vi "Main.vi"() -> ()   [LabVIEW 2018] (continued)
                n1556 = property on="102" class="Bool (严格)"("Colors [4]"=w7382) -> ()  [unwired: 2 in, 2 out]
                n1557 = property on="201" class="Bool (严格)"("Colors [4]"=w7382) -> ()  [unwired: 2 in, 2 out]
                n1558 = property on="301" class="Bool (严格)"("Colors [4]"=w7382) -> ()  [unwired: 2 in, 2 out]
                n1559 = property on="401" class="Bool (严格)"("Colors [4]"=w7382) -> ()  [unwired: 2 in, 2 out]
                n1560 = property on="501" class="Bool (严格)"("Colors [4]"=w7382) -> ()  [unwired: 2 in, 2 out]
                n1561 = property on="502" class="Bool (严格)"("Colors [4]"=w7382) -> ()  [unwired: 2 in, 2 out]
                n1562 = property on="503" class="Bool (严格)"("Colors [4]"=w7382) -> ()  [unwired: 2 in, 2 out]
                n1563 = property on="601" class="Bool (严格)"("Colors [4]"=w7382) -> ()  [unwired: 2 in, 2 out]
                n1564 = property on="70" class="Bool (严格)"("Colors [4]"=w7382) -> ()  [unwired: 2 in, 2 out]
                n1565 = property on="80" class="Bool (严格)"("Colors [4]"=w7382) -> ()  [unwired: 2 in, 2 out]
                n1566 = property on="901" class="Bool (严格)"("Colors [4]"=w7382) -> ()  [unwired: 2 in, 2 out]
                n1567 = property on="902" class="Bool (严格)"("Colors [4]"=w7382) -> ()  [unwired: 2 in, 2 out]
                n1568 = property on="602" class="Bool (严格)"("Colors [4]"=w7382) -> ()  [unwired: 2 in, 2 out]
                n1569 = property on="603" class="Bool (严格)"("Colors [4]"=w7382) -> ()  [unwired: 2 in, 2 out]
                n1570 = property on="202" class="Bool (严格)"("Colors [4]"=w7382) -> ()  [unwired: 2 in, 2 out]
                n1571 = property on="302" class="Bool (严格)"("Colors [4]"=w7382) -> ()  [unwired: 2 in, 2 out]
                n1572 = property on="303" class="Bool (严格)"("Colors [4]"=w7382) -> ()  [unwired: 2 in, 2 out]
                n1573 = property on="402" class="Bool (严格)"("Colors [4]"=w7382) -> ()  [unwired: 2 in, 2 out]
                n1574 = property on="504" class="Bool (严格)"("Colors [4]"=w7382) -> ()  [unwired: 2 in, 2 out]
              }
              frame #1 {
                n1575 = Concatenate Strings("Where QRCode='" ("查询语句"), "输入需要Rework的一维码：", "'" ("字符串")) -> (w7412:string)
                n1576 = call "SQL_Select.vi"("要读取的列名"=string[] ["Last_Station", "Last_Result"] ("列名"), "表名"="Online", "error in (no error)"=w7410, "查询语句"=w7412, "查询条件"=TRUE, "connection reference"=w7411) -> ("error out"=w7402:errorcluster, "数据"=w7407:string[][])  [unwired: 3 in, 1 out]
                n1577 = Index Array(array=w7407, index (row)=0 ("索引 (行)")) -> (element=w7405:string[])  [unwired: 1 in]
                n1578 = Index Array(array=w7405) -> (element #1=w7404:string, element #2=w7403:string)  [unwired: 2 in]
                n1579 = case shown="\"902\"" w7404 {
                  tunnel: [w7417 w7419 TRUE w7432 w7439 w7446 w7453 w7460 w7467 w7474 w7481 w7488 w7495 w7502 w7509 w7516 w7523 w7530 w7537 w7543] -> w7401
                  tunnel: [w7417 w7418 w7426 w7432 w7439 w7446 w7453 w7460 w7467 w7474 w7481 w7488 w7495 w7502 w7509 w7516 w7523 w7530 w7537 w7543] -> w7400
                  tunnel: [w7417 w7418 w7424 w7433 w7439 w7446 w7453 w7460 w7467 w7474 w7481 w7488 w7495 w7502 w7509 w7516 w7523 w7530 w7537 w7543] -> w7399
                  tunnel: [w7417 w7418 w7424 w7431 w7440 w7446 w7453 w7460 w7467 w7474 w7481 w7488 w7495 w7502 w7509 w7516 w7523 w7530 w7537 w7543] -> w7398
                  tunnel: [w7417 w7418 w7424 w7431 w7438 w7447 w7453 w7460 w7467 w7474 w7481 w7488 w7495 w7502 w7509 w7516 w7523 w7530 w7537 w7543] -> w7397
                  tunnel: [w7417 w7418 w7424 w7431 w7438 w7445 w7454 w7460 w7467 w7474 w7481 w7488 w7495 w7502 w7509 w7516 w7523 w7530 w7537 w7543] -> w7396
                  tunnel: [w7417 w7418 w7424 w7431 w7438 w7445 w7452 w7461 w7467 w7474 w7481 w7488 w7495 w7502 w7509 w7516 w7523 w7530 w7537 w7543] -> w7395
                  tunnel: [w7417 w7418 w7424 w7431 w7438 w7445 w7452 w7459 w7468 w7474 w7481 w7488 w7495 w7502 w7509 w7516 w7523 w7530 w7537 w7543] -> w7394
                  tunnel: [w7417 w7418 w7424 w7431 w7438 w7445 w7452 w7459 w7466 w7475 w7481 w7488 w7495 w7502 w7509 w7516 w7523 w7530 w7537 w7543] -> w7393
                  tunnel: [w7417 w7418 w7424 w7431 w7438 w7445 w7452 w7459 w7466 w7473 w7483 w7488 w7495 w7502 w7509 w7516 w7523 w7530 w7537 w7543] -> w7392
                  tunnel: [w7417 w7418 w7424 w7431 w7438 w7445 w7452 w7459 w7466 w7473 w7480 w7490 w7495 w7502 w7509 w7516 w7523 w7530 w7537 w7543] -> w7391
                  tunnel: [w7417 w7418 w7424 w7431 w7438 w7445 w7452 w7459 w7466 w7473 w7480 w7487 w7496 w7502 w7509 w7516 w7523 w7530 w7537 w7543] -> w7390
                  tunnel: [w7417 w7418 w7424 w7431 w7438 w7445 w7452 w7459 w7466 w7473 w7480 w7487 w7494 w7504 w7509 w7516 w7523 w7530 w7537 w7543] -> w7389
                  tunnel: [w7417 w7418 w7424 w7431 w7438 w7445 w7452 w7459 w7466 w7473 w7480 w7487 w7494 w7501 w7510 w7516 w7523 w7530 w7537 w7543] -> w7388
                  tunnel: [w7417 w7418 w7424 w7431 w7438 w7445 w7452 w7459 w7466 w7473 w7480 w7487 w7494 w7501 w7508 w7517 w7523 w7530 w7537 w7543] -> w7387
                  tunnel: [w7417 w7418 w7424 w7431 w7438 w7445 w7452 w7459 w7466 w7473 w7480 w7487 w7494 w7501 w7508 w7515 w7524 w7530 w7537 w7543] -> w7386
                  tunnel: [w7417 w7418 w7424 w7431 w7438 w7445 w7452 w7459 w7466 w7473 w7480 w7487 w7494 w7501 w7508 w7515 w7522 w7531 w7537 w7543] -> w7385
                  tunnel: [w7417 w7418 w7424 w7431 w7438 w7445 w7452 w7459 w7466 w7473 w7480 w7487 w7494 w7501 w7508 w7515 w7522 w7529 w7539 w7543] -> w7384
                  tunnel: [w7417 w7418 w7424 w7431 w7438 w7445 w7452 w7459 w7466 w7473 w7480 w7487 w7494 w7501 w7508 w7515 w7522 w7529 FALSE w7545] -> w7383
                  tunnel: w7403 -> [_ w7420 w7427 w7434 w7441 w7448 w7455 w7462 w7469 w7476 w7482 w7489 w7497 w7503 w7511 w7518 w7525 w7532 w7538 w7544]
                  frame "0", Default {
                    w7417 = FALSE
                  }
                  frame "102" {
                    w7418 = FALSE
                    n1580 = case shown="\"NG\"" w7420 {
                      tunnel: [TRUE FALSE] -> w7419
                      frame "OK", Default {
                      }
                      frame "NG" {
                        n1581 = property on="102" class="Bool (严格)"("Colors [4]"=cluster{u32, u32}[] [{16711680, 16711680}, {6618880, 6618880}, {1985280, 1985280}, {6618880, 6618880}] ("颜色[4]")) -> ()  [unwired: 2 in, 2 out]
                      }
                    }
                  }
                  frame "201" {
                    w7424 = FALSE
                    n1582 = case shown="\"NG\"" w7427 {
                      tunnel: [TRUE FALSE] -> w7426
                      frame "OK", Default {
                      }
                      frame "NG" {
                        n1583 = property on="201" class="Bool (严格)"("Colors [4]"=cluster{u32, u32}[] [{16711680, 16711680}, {6618880, 6618880}, {1985280, 1985280}, {6618880, 6618880}] ("颜色[4]")) -> ()  [unwired: 2 in, 2 out]
                      }
                    }
                  }
                  frame "202" {
                    w7432 = TRUE
                    w7431 = FALSE
                    n1584 = case shown="\"NG\"" w7434 {
                      tunnel: [TRUE FALSE] -> w7433
                      frame "OK", Default {
                      }
                      frame "NG" {
                        n1585 = property on="202" class="Bool (严格)"("Colors [4]"=cluster{u32, u32}[] [{16711680, 16711680}, {6618880, 6618880}, {1985280, 1985280}, {6618880, 6618880}] ("颜色[4]")) -> ()  [unwired: 2 in, 2 out]
                      }
                    }
                  }
                  frame "301" {
                    w7438 = FALSE
                    w7439 = TRUE
                    n1586 = case shown="\"NG\"" w7441 {
                      tunnel: [TRUE FALSE] -> w7440
                      frame "OK", Default {
                      }
                      frame "NG" {
                        n1587 = property on="301" class="Bool (严格)"("Colors [4]"=cluster{u32, u32}[] [{16711680, 16711680}, {6618880, 6618880}, {1985280, 1985280}, {6618880, 6618880}] ("颜色[4]")) -> ()  [unwired: 2 in, 2 out]
                      }
                    }
                  }
                  frame "302" {
                    w7445 = FALSE
                    w7446 = TRUE
                    n1588 = case shown="\"NG\"" w7448 {
                      tunnel: [TRUE FALSE] -> w7447
                      frame "OK", Default {
                      }
                      frame "NG" {
                        n1589 = property on="302" class="Bool (严格)"("Colors [4]"=cluster{u32, u32}[] [{16711680, 16711680}, {6618880, 6618880}, {1985280, 1985280}, {6618880, 6618880}] ("颜色[4]")) -> ()  [unwired: 2 in, 2 out]
                      }
                    }
                  }
                  frame "303" {
                    w7452 = FALSE
                    w7453 = TRUE
                    n1590 = case shown="\"NG\"" w7455 {
                      tunnel: [TRUE FALSE] -> w7454
                      frame "OK", Default {
                      }
                      frame "NG" {
                        n1591 = property on="303" class="Bool (严格)"("Colors [4]"=cluster{u32, u32}[] [{16711680, 16711680}, {6618880, 6618880}, {1985280, 1985280}, {6618880, 6618880}] ("颜色[4]")) -> ()  [unwired: 2 in, 2 out]
                      }
                    }
                  }
                  frame "401" {
                    w7459 = FALSE
                    w7460 = TRUE
                    n1592 = case shown="\"NG\"" w7462 {
                      tunnel: [TRUE FALSE] -> w7461
                      frame "OK", Default {
                      }
                      frame "NG" {
                        n1593 = property on="401" class="Bool (严格)"("Colors [4]"=cluster{u32, u32}[] [{16711680, 16711680}, {6618880, 6618880}, {1985280, 1985280}, {6618880, 6618880}] ("颜色[4]")) -> ()  [unwired: 2 in, 2 out]
                      }
                    }
                  }
                  frame "402" {
                    w7466 = FALSE
                    w7467 = TRUE
                    n1594 = case shown="\"NG\"" w7469 {
                      tunnel: [TRUE FALSE] -> w7468
                      frame "OK", Default {
                      }
                      frame "NG" {
                        n1595 = property on="402" class="Bool (严格)"("Colors [4]"=cluster{u32, u32}[] [{16711680, 16711680}, {6618880, 6618880}, {1985280, 1985280}, {6618880, 6618880}] ("颜色[4]")) -> ()  [unwired: 2 in, 2 out]
                      }
                    }
                  }
                  frame "501" {
                    w7473 = FALSE
                    w7474 = TRUE
                    n1596 = case shown="\"NG\"" w7476 {
                      tunnel: [TRUE FALSE] -> w7475
                      frame "OK", Default {
                      }
                      frame "NG" {
                        n1597 = property on="501" class="Bool (严格)"("Colors [4]"=cluster{u32, u32}[] [{16711680, 16711680}, {6618880, 6618880}, {1985280, 1985280}, {6618880, 6618880}] ("颜色[4]")) -> ()  [unwired: 2 in, 2 out]
                      }
                    }
                  }
                  frame "502" {
                    w7480 = FALSE
                    w7481 = TRUE
                    n1598 = case shown="\"NG\"" w7482 {
                      tunnel: [TRUE FALSE] -> w7483
                      frame "OK", Default {
                      }
                      frame "NG" {
                        n1599 = property on="502" class="Bool (严格)"("Colors [4]"=cluster{u32, u32}[] [{16711680, 16711680}, {6618880, 6618880}, {1985280, 1985280}, {6618880, 6618880}] ("颜色[4]")) -> ()  [unwired: 2 in, 2 out]
                      }
                    }
                  }
                  frame "503" {
                    w7487 = FALSE
                    w7488 = TRUE
                    n1600 = case shown="\"NG\"" w7489 {
                      tunnel: [TRUE FALSE] -> w7490
                      frame "OK", Default {
                      }
                      frame "NG" {
                        n1601 = property on="503" class="Bool (严格)"("Colors [4]"=cluster{u32, u32}[] [{16711680, 16711680}, {6618880, 6618880}, {1985280, 1985280}, {6618880, 6618880}] ("颜色[4]")) -> ()  [unwired: 2 in, 2 out]
                      }
                    }
                  }
                  frame "504" {
                    w7494 = FALSE
                    w7495 = TRUE
                    n1602 = case shown="\"NG\"" w7497 {
                      tunnel: [TRUE FALSE] -> w7496
                      frame "OK", Default {
                      }
                      frame "NG" {
                        n1603 = property on="504" class="Bool (严格)"("Colors [4]"=cluster{u32, u32}[] [{16711680, 16711680}, {6618880, 6618880}, {1985280, 1985280}, {6618880, 6618880}] ("颜色[4]")) -> ()  [unwired: 2 in, 2 out]
                      }
                    }
                  }
                  frame "601" {
                    w7501 = FALSE
                    w7502 = TRUE
                    n1604 = case shown="\"NG\"" w7503 {
                      tunnel: [TRUE FALSE] -> w7504
                      frame "OK", Default {
                      }
                      frame "NG" {
                        n1605 = property on="601" class="Bool (严格)"("Colors [4]"=cluster{u32, u32}[] [{16711680, 16711680}, {6618880, 6618880}, {1985280, 1985280}, {6618880, 6618880}] ("颜色[4]")) -> ()  [unwired: 2 in, 2 out]
                      }
                    }
                  }
                  frame "602" {
                    w7508 = FALSE
                    w7509 = TRUE
                    n1606 = case shown="\"NG\"" w7511 {
                      tunnel: [TRUE FALSE] -> w7510
                      frame "OK", Default {
                      }
                      frame "NG" {
                        n1607 = property on="602" class="Bool (严格)"("Colors [4]"=cluster{u32, u32}[] [{16711680, 16711680}, {6618880, 6618880}, {1985280, 1985280}, {6618880, 6618880}] ("颜色[4]")) -> ()  [unwired: 2 in, 2 out]
                      }
                    }
                  }
                  frame "603" {
                    w7515 = FALSE
                    w7516 = TRUE
                    n1608 = case shown="\"NG\"" w7518 {
                      tunnel: [TRUE FALSE] -> w7517
                      frame "OK", Default {
                      }
                      frame "NG" {
                        n1609 = property on="603" class="Bool (严格)"("Colors [4]"=cluster{u32, u32}[] [{16711680, 16711680}, {6618880, 6618880}, {1985280, 1985280}, {6618880, 6618880}] ("颜色[4]")) -> ()  [unwired: 2 in, 2 out]
                      }
                    }
                  }
                  frame "70" {
                    w7522 = FALSE
                    w7523 = TRUE
                    n1610 = case shown="\"NG\"" w7525 {
                      tunnel: [TRUE FALSE] -> w7524
                      frame "OK", Default {
                      }
                      frame "NG" {
                        n1611 = property on="70" class="Bool (严格)"("Colors [4]"=cluster{u32, u32}[] [{16711680, 16711680}, {6618880, 6618880}, {1985280, 1985280}, {6618880, 6618880}] ("颜色[4]")) -> ()  [unwired: 2 in, 2 out]
                      }
                    }
                  }
                  frame "80" {
                    w7529 = FALSE
                    w7530 = TRUE
                    n1612 = case shown="\"NG\"" w7532 {
                      tunnel: [TRUE FALSE] -> w7531
                      frame "OK", Default {
                      }
                      frame "NG" {
                        n1613 = property on="80" class="Bool (严格)"("Colors [4]"=cluster{u32, u32}[] [{16711680, 16711680}, {6618880, 6618880}, {1985280, 1985280}, {6618880, 6618880}] ("颜色[4]")) -> ()  [unwired: 2 in, 2 out]
                      }
                    }
                  }
                  frame "901" {
                    w7537 = TRUE
                    n1614 = case shown="\"OK\", 默认" w7538 {
                      tunnel: [TRUE FALSE] -> w7539
                      frame "OK", Default {
                      }
                      frame "NG" {
                        n1615 = property on="901" class="Bool (严格)"("Colors [4]"=cluster{u32, u32}[] [{16711680, 16711680}, {6618880, 6618880}, {1985280, 1985280}, {6618880, 6618880}] ("颜色[4]")) -> ()  [unwired: 2 in, 2 out]
                      }
                    }
                  }
                  frame "902" {
                    w7543 = TRUE
                    n1616 = case shown="\"NG\"" w7544 {
                      tunnel: [TRUE FALSE] -> w7545
                      frame "OK", Default {
                      }
                      frame "NG" {
                        n1617 = property on="902" class="Bool (严格)"("Colors [4]"=cluster{u32, u32}[] [{16711680, 16711680}, {6618880, 6618880}, {1985280, 1985280}, {6618880, 6618880}] ("颜色[4]")) -> ()  [unwired: 2 in, 2 out]
                      }
                    }
                  }
                }
                n1618 = local write "102"(w7401) -> ()
                n1619 = local write "201"(w7400) -> ()
                n1620 = local write "202"(w7399) -> ()
                n1621 = local write "301"(w7398) -> ()
                n1622 = local write "302"(w7397) -> ()
                n1623 = local write "303"(w7396) -> ()
                n1624 = local write "401"(w7395) -> ()
                n1625 = local write "402"(w7394) -> ()
                n1626 = local write "501"(w7393) -> ()
                n1627 = local write "502"(w7392) -> ()
                n1628 = local write "503"(w7391) -> ()
                n1629 = local write "504"(w7390) -> ()
                n1630 = local write "601"(w7389) -> ()
                n1631 = local write "602"(w7388) -> ()
                n1632 = local write "603"(w7387) -> ()
                n1633 = local write "70"(w7386) -> ()
                n1634 = local write "80"(w7385) -> ()
                n1635 = local write "901"(w7384) -> ()
                n1636 = local write "902"(w7383) -> ()
              }
            }
          }
          event "确定Rework": Value Change {
            n1637 = event-data() -> ()  [unwired: 1 in, 2 out]
            n1638 = stacked-sequence {
              seq-local: [w7553 _] -> [_ w7586]
              tunnel: w7552 -> [w7563 w7591]
              tunnel: w7551 -> [w7562 w7590]
              tunnel: [_ w7589] -> w7550
              frame #0 {
                n1639 = local read "输入需要Rework的一维码："() -> (w7558:string)
                n1640 = Concatenate Strings("Where QRCode='" ("查询语句"), w7558, "'" ("字符串")) -> (w7557:string)
                n1641 = call "SQL_Select.vi"("表名"="Online", "error in (no error)"=w7562, "查询语句"=w7557, "查询条件"=TRUE, "connection reference"=w7563) -> ("数据"=w7556:string[][])  [unwired: 4 in, 2 out]
                n1642 = Matrix Size(0:w7556) -> (1:w7555:i32)  [unwired: 1 out]
                n1643 = Equal?(x=w7555, y=0) -> (x = y?=w7553:bool)
              }
              frame #1 {
                n1644 = Insert Into Array(array=bool[] [] ("数组"), index=0 ("索引"), new element #1="902", new element #2="901", new element #3="80", new element #4="70", new element #5="603", new element #6="602", new element #7="601", new element #8="504", new element #9="503", new element #10="502", new element #11="501", new element #12="402", new element #13="401", new element #14="303", new element #15="302", new element #16="301", new element #17="202", new element #18="201", new element #19="102") -> (w7595:bool[])
                n1645 = Search 1D Array(1D array=w7595, element=TRUE ("元素")) -> (index of element=w7592:i32)  [unwired: 1 in]
                n1646 = Equal?(x=w7592, y=-1) -> (x = y?=w7588:bool)
                n1647 = Or(x=w7588, y=w7586) -> (x .or. y?=w7587:bool)
                n1648 = case shown="假" w7587 {
                  tunnel: w7592 -> [w7637 _]
                  tunnel: w7591 -> [w7636 _]
                  tunnel: w7590 -> [w7635 w7754]
                  tunnel: [w7597 w7754] -> w7589
                  frame False {
                    w7609 = "Rework_List" ("表名")
                    w7607 = 0 ("索引 (行)")
                    w7620 = "Online" ("表名")
                    n1649 = case shown="8" w7637 {
                      tunnel: w7636 -> [w7698 w7700 w7704 w7707 w7710 w7713 w7716 w7719 w7722 w7725 w7728 w7731 w7733 w7736 w7739 w7742 w7745 w7748 w7751]
                      tunnel: w7635 -> [w7697 w7699 w7703 w7706 w7709 w7712 w7715 w7718 w7721 w7724 w7727 w7730 w7732 w7735 w7738 w7741 w7744 w7747 w7750]
                      tunnel: [w7697 w7699 w7703 w7706 w7709 w7712 w7715 w7718 w7721 w7724 w7727 w7730 w7732 w7735 w7738 w7741 w7744 w7747 w7750] -> w7623
                      tunnel: [w7698 w7700 w7704 w7707 w7710 w7713 w7716 w7719 w7722 w7725 w7728 w7731 w7733 w7736 w7739 w7742 w7745 w7748 w7751] -> w7624
                      tunnel: ["902" "901" "80" "70" "603" "602" "601" "504" "503" "502" "501" "402" "401" "303" "302" "301" "202" "201" "102"] -> w7604
                      frame 0, Default {
                      }
                      frame 1 {
                      }
                      frame 2 {
                      }
                      frame 3 {
                      }
                      frame 4 {
                      }
                      frame 5 {
                      }
                      frame 6 {
                      }
                      frame 7 {
                      }
                      frame 8 {
                      }
                      frame 9 {
                      }
                      frame 10 {
                      }
                      frame 11 {
                      }
                      frame 12 {
                      }
                      frame 13 {
                      }
                      frame 14 {
                      }
                      frame 15 {
                      }
                      frame 16 {
                      }
                      frame 17 {
                      }
                      frame 18 {
                      }
                    }
                    n1650 = local read "输入需要Rework的一维码："() -> (w7599:string)
                    n1651 = Concatenate Strings("Where QRCode='" ("查询语句"), w7599, "'" ("字符串")) -> (w7606:string)
                    n1652 = call "SQL_Select.vi"("要读取的列名"=string[] ["Last_Station"], "表名"=w7620, "error in (no error)"=w7623, "查询语句"=w7606, "查询条件"=TRUE, "connection reference"=w7624) -> ("error out"=w7621:errorcluster, "数据"=w7596:string[][], "connection reference out"=w7622:T5)  [unwired: 3 in]
                    n1653 = Index Array(array=w7596, index (row)=w7607, index (col)=w7607) -> (element=w7605:string)
                    n1654 = Insert Into Array(array=string[] [] ("数组"), index=0 ("索引"), new element #1=w7604, new element #2="OK" ("新元素/子数组"), new element #3="T" ("新元素/子数组")) -> (w7633:string[])
                    n1655 = call "SQL_Update.vi"("查询语句"=w7606, "表名"=w7620, "error in (no error)"=w7621, "列名对应的值"=w7633, "列名"=string[] ["Last_Station", "Last_Result", "Rework_Status"], "connection reference"=w7622) -> ("error out"=w7619:errorcluster, "connection reference 2"=w7618:T5)  [unwired: 4 in]
                    n1656 = call "SQL_Select.vi"("表名"=w7609, "error in (no error)"=w7619, "查询语句"=w7606, "查询条件"=TRUE, "connection reference"=w7618) -> ("error out"=w7612:errorcluster, "数据"=w7616:string[][], "connection reference out"=w7613:T5)  [unwired: 4 in]
                    n1657 = Matrix Size(0:w7616) -> (1:w7615:i32)  [unwired: 1 out]
                    n1658 = call "Rework_Calculate.vi"("Rework站号"=w7604, "当前站号"=w7605) -> ("Data"=w7611:string[], "Rework_List"=w7610:string[], "跨站"=w7603:bool)  [unwired: 7 in]
                    n1659 = Equal To 0?(x=w7615) -> (x = 0?=w7614:bool)
                    n1660 = case shown="假" w7603 {
                      tunnel: w7614 -> [w7656 _]
                      tunnel: w7613 -> [w7655 w7692]
                      tunnel: w7612 -> [w7654 w7693]
                      tunnel: w7611 -> [w7653 _]
                      tunnel: w7610 -> [w7652 _]
                      tunnel: w7609 -> [w7651 _]
                      tunnel: w7606 -> [w7647 _]
                      tunnel: w7599 -> [w7640 _]
                      tunnel: [w7639 w7693] -> w7601
                      tunnel: [w7638 w7692] -> w7602
                      frame False {
                        w7641 = "Rework" ("表名")
                        n1661 = case shown="真" w7656 {
                          tunnel: w7655 -> [w7678 w7691]
                          tunnel: w7654 -> [w7677 w7690]
                          tunnel: w7653 -> [w7675 w7685]
                          tunnel: w7652 -> [w7676 w7688]
                          tunnel: w7651 -> [w7674 w7689]
                          tunnel: w7640 -> [_ w7683]
                          tunnel: [w7672 w7680] -> w7649
                          tunnel: [w7671 w7679] -> w7648
                          tunnel: w7647 -> [w7673 _]
                          frame False {
                            n1662 = call "SQL_Update.vi"("查询语句"=w7673, "表名"=w7674, "error in (no error)"=w7677, "列名对应的值"=w7675, "列名"=w7676, "connection reference"=w7678) -> ("error out"=w7671:errorcluster, "connection reference 2"=w7672:T5)  [unwired: 4 in]
                          }
                          frame True {
                            n1663 = Insert Into Array(array=w7688, index=0 ("索引"), new element="QRCode" ("新元素/子数组")) -> (w7682:string[])
                            n1664 = Insert Into Array(array=w7685, index=0 ("索引"), new element=w7683) -> (w7681:string[])
                            n1665 = call "SQL_Insert.vi"("表名"=w7689, "error in (no error)"=w7690, "值"=w7681, "列名"=w7682, "connection reference"=w7691) -> ("error out"=w7679:errorcluster, "connection reference 2"=w7680:T5)  [unwired: 5 in]
                          }
                        }
                        n1666 = call "SQL_Select.vi"("表名"=w7641, "error in (no error)"=w7648, "查询语句"=w7647, "查询条件"=TRUE, "connection reference"=w7649) -> ("error out"=w7642:errorcluster, "数据"=w7646:string[][], "connection reference out"=w7643:T5)  [unwired: 4 in]
                        n1667 = Matrix Size(0:w7646) -> (1:w7645:i32)  [unwired: 1 out]
                        n1668 = Equal To 0?(x=w7645) -> (x = 0?=w7644:bool)
                        n1669 = case shown="真" w7644 {
                          tunnel: w7643 -> [w7657 w7670]
                          tunnel: w7642 -> [w7658 w7669]
                          tunnel: w7641 -> [_ w7668]
                          tunnel: w7640 -> [_ w7666]
                          tunnel: [w7658 w7662] -> w7639
                          tunnel: [w7657 w7659] -> w7638
                          frame False {
                          }
                          frame True {
                            n1670 = Format Date/Time String(time format string (%c)="%Y-%m-%d_%H:%M" ("时间格式字符串(%c)")) -> (date/time string=w7660:string)  [unwired: 2 in]
                            n1671 = Insert Into Array(array=string[] [] ("数组"), index=0 ("索引"), new element #1=w7666, new element #2=w7660) -> (w7663:string[])
                            n1672 = call "SQL_Insert.vi"("表名"=w7668, "error in (no error)"=w7669, "值"=w7663, "列名"=string[] ["QRCode", "Online_Time"], "connection reference"=w7670) -> ("error out"=w7662:errorcluster, "connection reference 2"=w7659:T5)  [unwired: 5 in]
                          }
                        }
                      }
                      frame True {
                      }
                    }
                    n1673 = call "SQL_Delete.vi"("表名"="Time", "error in (no error)"=w7601, "值"=w7599, "列名"="QRCode", "connection reference"=w7602) -> ("error out"=w7597:errorcluster)  [unwired: 5 in, 1 out]
                    n1674 = case shown="错误" w7597 {
                      tunnel: ["Rework成功！" ("Rework状态") "Rework失败！" ("Rework状态")] -> w7608
                      frame No Error {
                      }
                      frame Error {
                      }
                    }
                    "Rework状态" <- w7608
                  }
                  frame True {
                    n1675 = local write "Rework状态"("该条码不存在！" ("Rework状态")) -> ()
                  }
                }
              }
            }
          }
        }
        n1676 = case shown="错误" w4418 {
          selector: w4418 -> [_ w4425]
          tunnel: w4417 -> [_ w4430]
          frame No Error {
          }
          frame Error {
            n1677 = Unbundle By Name(w4425) -> ("source"=w4424:string)
            n1678 = property on="错误信息" class="LstBox (严格)"() -> ("Item Names"=w4429:string[])  [unwired: 2 in, 2 out]
            n1679 = Format Date/Time String(time format string (%c)="%Y-%m-%d %H:%M:%S" ("时间格式字符串(%c)")) -> (date/time string=w4432:string)  [unwired: 2 in]
            n1680 = Concatenate Strings(w4432, "  " ("字符串"), w4430, w4424) -> (w4427:string)
            n1681 = Insert Into Array(array=w4429, index=0 ("索引"), new element=w4427) -> (w4426:string[])
            n1682 = property on="错误信息" class="LstBox (严格)"("Item Names"=w4426) -> ()  [unwired: 2 in, 2 out]
          }
        }
        n1683 = local read "退出"() -> (w4419:bool)
        n1684 = Wait (ms)(milliseconds to wait=u32 30 ("等待时间（毫秒）")) -> ()  [unwired: 1 out]
      }
      n1685 = while {
        shift-right: [w4049] -> _
        shift-left: errorcluster {"status"=FALSE, "code"=0, "source"=""} ("错误常量") -> [w4052]
        shift-right: [w4048] -> _
        shift-left: enum16{"初始化", "读", "写", "错误", "退出"}."初始化" -> [w4054]
        shift-right: [w4050] -> _
        shift-left: _ -> [w4046]
        stop <- w4047 stop-if-true
        # "原100"
        n1686 = local read "退出"() -> (w4055:bool)
        n1687 = case shown="假" w4055 {
          tunnel: w4054 -> [w4056 _]
          tunnel: [w4057 enum16{"初始化", "读", "写", "错误", "退出"}."退出"] -> w4053
          tunnel: w4052 -> [w4058 _]
          frame False {
            n1688 = case shown="错误" w4058 {
              tunnel: [w4059 enum16{"初始化", "读", "写", "错误", "退出"}."错误"] -> w4057
              tunnel: w4056 -> [w4059 _]
              frame No Error {
              }
              frame Error {
              }
            }
          }
          frame True {
          }
        }
        n1689 = Wait (ms)(milliseconds to wait=u32 20 ("等待时间（毫秒）")) -> ()  [unwired: 1 out]
        n1690 = case shown="\"写\"" w4053 {
          tunnel: [w4065 w4104 w4311 refnum<k5> refnum ("TCP") refnum<k5> refnum ("TCP")] -> w4050
          tunnel: [w4063 w4103 w4313 errorcluster {"status"=FALSE, "code"=0, "source"=""} ("error out") errorcluster {"status"=FALSE, "code"=0, "source"=""} ("error out")] -> w4049
          tunnel: [enum16{"初始化", "读", "写", "错误", "退出"}."读" enum16{"初始化", "读", "写", "错误", "退出"}."写" enum16{"初始化", "读", "写", "错误", "退出"}."读" enum16{"初始化", "读", "写", "错误", "退出"}."初始化" enum16{"初始化", "读", "写", "错误", "退出"}."退出"] -> w4048
          tunnel: w4046 -> [_ w4145 w4342 w4407 w4414]
          tunnel: [FALSE FALSE FALSE FALSE TRUE] -> w4047
          frame "初始化", Default {
            w4066 = u16 0 items=["byte", "word", "Dword"] ("数据类型")
            w4068 = u8 132 items=["I/O (P)"=128, "Input (I)"=129, "Output (Q)"=130, "Bit Memory (M)"=131, "Data (DB)"=132, "Instance Data (DI)"=133, "Local Data (L)"=134, "Predecessor Local Data (VL)"=135] ("寄存器类型")
            w4082 = u16 0 items=["byte", "word", "Dword"] ("数据类型")
            w4084 = u8 132 items=["I/O (P)"=128, "Input (I)"=129, "Output (Q)"=130, "Bit Memory (M)"=131, "Data (DB)"=132, "Instance Data (DI)"=133, "Local Data (L)"=134, "Predecessor Local Data (VL)"=135] ("寄存器类型")
            w4091 = u8 0 items=["S7-1200.200.200SMART"=0, "S7-300"=2, "S7-400"=3] ("PLC 系列")
            n1691 = call "S7_Open.vi"("IP 地址"="192.168.1.10", "PLC 系列"=w4091, "超时（MS）"=100) -> ("TCP"=w4081:refnum<k5>, "error out"=w4080:errorcluster)  [unwired: 10 in, 1 out]
            n1692 = case shown="错误" w4080 {
              tunnel: [FALSE TRUE] -> w4087
              frame No Error {
              }
              frame Error {
              }
            }
            n1693 = local write "ST10通讯状态"(w4087) -> ()
            n1694 = call "S7_Read.vi"("TCP"=w4081, "DB #"=u16 20, "读取长度"=u16 15, "寄存器类型"=w4084, "起始地址"=u32 14, "数据类型"=w4082, "error in"=w4080) -> ("TCP"=w4065:refnum<k5>, "数据"=w4079:u32[], "error out"=w4064:errorcluster)  [unwired: 5 in, 1 out]
            n1695 = Delete From Array(array=w4079, length=2 ("长度"), index=0 ("索引")) -> (array with subset deleted=w4076:u32[])  [unwired: 1 out]
            n1696 = To Unsigned Byte Integer(number=w4076) -> (unsigned 8bit integer=w4075:u8[])
            n1697 = Byte Array To String(unsigned byte array=w4075) -> (string=w4074:string)
            n1698 = local write "101二维码"(w4074) -> ()
            n1699 = call "S7_Read.vi"("TCP"=w4065, "DB #"=u16 20, "读取长度"=u16 13, "寄存器类型"=w4068, "起始地址"=u32 38, "数据类型"=w4066, "error in"=w4064) -> ("数据"=w4071:u32[], "error out"=w4073:errorcluster)  [unwired: 5 in, 2 out]
            n1700 = To Unsigned Word Integer(number=w4071) -> (unsigned 16bit integer=w4072:u16[])
            n1701 = call "还原为字符串.vi"("error in (no error)"=w4073, "输入数组"=w4072) -> ("error out"=w4063:errorcluster, "字符串"=w4062:string)  [unwired: 8 in]
            n1702 = local write "102二维码"(w4062) -> ()
          }
          frame "读" {
            w4114 = u16 0 items=["byte", "word", "Dword"] ("数据类型")
            w4116 = u8 132 items=["I/O (P)"=128, "Input (I)"=129, "Output (Q)"=130, "Bit Memory (M)"=131, "Data (DB)"=132, "Instance Data (DI)"=133, "Local Data (L)"=134, "Predecessor Local Data (VL)"=135] ("寄存器类型")
            w4107 = u16 0 items=["byte", "word", "Dword"] ("数据类型")
            w4109 = u8 132 items=["I/O (P)"=128, "Input (I)"=129, "Output (Q)"=130, "Bit Memory (M)"=131, "Data (DB)"=132, "Instance Data (DI)"=133, "Local Data (L)"=134, "Predecessor Local Data (VL)"=135] ("寄存器类型")
            w4146 = u16 0 items=["byte", "word", "Dword"] ("数据类型")
            w4148 = u8 132 items=["I/O (P)"=128, "Input (I)"=129, "Output (Q)"=130, "Bit Memory (M)"=131, "Data (DB)"=132, "Instance Data (DI)"=133, "Local Data (L)"=134, "Predecessor Local Data (VL)"=135] ("寄存器类型")
            n1703 = call "S7_Read.vi"("TCP"=w4145, "DB #"=u16 20, "读取长度"=u16 1, "寄存器类型"=w4148, "起始地址"=u32 0, "数据类型"=w4146) -> ("TCP"=w4143:refnum<k5>, "数据"=w4153:u32[], "读取成功"=w4095:bool, "error out"=w4142:errorcluster)  [unwired: 6 in]
            n1704 = Index Array(array=w4153, index=0 ("索引")) -> (element=w4154:u32)
            n1705 = Not(x=w4095) -> (.not. x?=→"ST10通讯状态":bool)
            n1706 = Number To Boolean Array(number=w4154) -> (Boolean array=w4155:bool[])
            n1707 = Index Array(array=w4155, index #1=0 ("索引")) -> (element #1=w4102:bool, element #2=w4099:bool, element #3=w4097:bool)  [unwired: 2 in]
            "ST101扫码请求" <- w4102
            "ST102扫码请求" <- w4099
            "ST102数据读取" <- w4097
            n1708 = disable-structure shown="启用" {
              disable-tunnel: w4102 -> [w4163 w4165]
              disable-tunnel: [w4162 w4165] -> w4101
              frame Disabled {
                n1709 = call <vilib>:"Boolean Crossing PtByPt.vi"("direction"=enum16{"either", "false-true", "true-false"}."true-false", "input"=w4163) -> ("crossing"=w4162:bool)  [unwired: 1 in]
              }
              frame Enabled {
              }
            }
            n1710 = call <vilib>:"Boolean Crossing PtByPt.vi"("direction"=enum16{"either", "false-true", "true-false"}."false-true", "input"=w4102) -> ("crossing"=w4141:bool)  [unwired: 1 in]
            n1711 = case shown="真" w4141 {
              tunnel: w4143 -> [w4281 w4287]
              tunnel: w4142 -> [w4280 w4286]
              tunnel: [w4281 w4285] -> w4140
              tunnel: [w4280 w4283] -> w4139
              frame False {
              }
              frame True {
                w4293 = u16 0 items=["byte", "word", "Dword"] ("数据类型")
                w4295 = u8 132 items=["I/O (P)"=128, "Input (I)"=129, "Output (Q)"=130, "Bit Memory (M)"=131, "Data (DB)"=132, "Instance Data (DI)"=133, "Local Data (L)"=134, "Predecessor Local Data (VL)"=135] ("寄存器类型")
                w4288 = u16 0 items=["byte", "word", "Dword"] ("数据类型")
                w4290 = u8 132 items=["I/O (P)"=128, "Input (I)"=129, "Output (Q)"=130, "Bit Memory (M)"=131, "Data (DB)"=132, "Instance Data (DI)"=133, "Local Data (L)"=134, "Predecessor Local Data (VL)"=135] ("寄存器类型")
                n1712 = call "S7_Read.vi"("TCP"=w4287, "DB #"=u16 20, "读取长度"=u16 1, "寄存器类型"=w4295, "起始地址"=u32 58, "数据类型"=w4293, "error in"=w4286) -> ("TCP"=w4299:refnum<k5>, "数据"=w4303:u32[], "error out"=w4301:errorcluster)  [unwired: 5 in, 1 out]
                n1713 = To Unsigned Word Integer(number=w4303) -> (unsigned 16bit integer=w4302:u16[])
                n1714 = call "还原为字符串.vi"("error in (no error)"=w4301, "输入数组"=w4302) -> ("error out"=w4300:errorcluster, "字符串"=→"101打码等级":string)  [unwired: 8 in]
                n1715 = call "S7_Read.vi"("TCP"=w4299, "DB #"=u16 20, "读取长度"=u16 13, "寄存器类型"=w4290, "起始地址"=u32 16, "数据类型"=w4288, "error in"=w4300) -> ("TCP"=w4285:refnum<k5>, "数据"=w4304:u32[], "error out"=w4306:errorcluster)  [unwired: 5 in, 1 out]
                n1716 = To Unsigned Word Integer(number=w4304) -> (unsigned 16bit integer=w4305:u16[])
                n1717 = call "还原为字符串.vi"("error in (no error)"=w4306, "输入数组"=w4305) -> ("error out"=w4284:errorcluster, "字符串"=w4282:string)  [unwired: 8 in]
                n1718 = stacked-sequence {
                  tunnel: w4284 -> [_ w4310]
                  tunnel: [_ w4308] -> w4283
                  tunnel: w4282 -> [w4307 _]
                  frame #0 {
                    "101二维码" <- w4307
                  }
                  frame #1 {
                    n1719 = property on="ST101扫码请求（事件）" class="Bool (严格)"(error in=w4310, "Val(Sgnl)"=TRUE ("值(信号)")) -> (error out=w4308:errorcluster)  [unwired: 1 in, 1 out]
                  }
                }
              }
            }
            n1720 = case shown="假" w4101 {
              frame False {
                n1721 = local write "101扫码回复写入"(FALSE ("101扫码回复写入")) -> ()
              }
              frame True {
              }
            }
            n1722 = disable-structure shown="启用" {
              disable-tunnel: [w4159 w4161] -> w4100
              disable-tunnel: w4099 -> [w4158 w4161]
              frame Disabled {
                n1723 = call <vilib>:"Boolean Crossing PtByPt.vi"("direction"=enum16{"either", "false-true", "true-false"}."true-false", "input"=w4158) -> ("crossing"=w4159:bool)  [unwired: 1 in]
              }
              frame Enabled {
              }
            }
            n1724 = call <vilib>:"Boolean Crossing PtByPt.vi"("direction"=enum16{"either", "false-true", "true-false"}."false-true", "input"=w4099) -> ("crossing"=w4137:bool)  [unwired: 1 in]
            n1725 = case shown="假" w4100 {
              frame False {
                n1726 = local write "102扫码回复写入"(FALSE ("102扫码回复写入")) -> ()
              }
              frame True {
              }
            }
            n1727 = case shown="真" w4137 {
              tunnel: [w4261 w4267] -> w4133
              tunnel: [w4260 w4263] -> w4134
              tunnel: w4139 -> [w4260 w4266]
              tunnel: w4140 -> [w4261 w4265]
              frame False {
              }
              frame True {
                w4268 = u16 0 items=["byte", "word", "Dword"] ("数据类型")
                w4270 = u8 132 items=["I/O (P)"=128, "Input (I)"=129, "Output (Q)"=130, "Bit Memory (M)"=131, "Data (DB)"=132, "Instance Data (DI)"=133, "Local Data (L)"=134, "Predecessor Local Data (VL)"=135] ("寄存器类型")
                n1728 = call "S7_Read.vi"("TCP"=w4265, "DB #"=u16 20, "读取长度"=u16 13, "寄存器类型"=w4270, "起始地址"=u32 38, "数据类型"=w4268, "error in"=w4266) -> ("TCP"=w4267:refnum<k5>, "数据"=w4273:u32[], "error out"=w4275:errorcluster)  [unwired: 5 in, 1 out]
                n1729 = To Unsigned Word Integer(number=w4273) -> (unsigned 16bit integer=w4274:u16[])
                n1730 = call "还原为字符串.vi"("error in (no error)"=w4275, "输入数组"=w4274) -> ("error out"=w4264:errorcluster, "字符串"=w4262:string)  [unwired: 8 in]
                n1731 = stacked-sequence {
                  tunnel: w4264 -> [_ w4278]
                  tunnel: [_ w4277] -> w4263
                  tunnel: w4262 -> [w4276 _]
                  frame #0 {
                    "102二维码" <- w4276
                  }
                  frame #1 {
                    n1732 = property on="ST102右扫码请求（事件）" class="Bool (严格)"(error in=w4278, "Val(Sgnl)"=TRUE ("值(信号)")) -> (error out=w4277:errorcluster)  [unwired: 1 in, 1 out]
                  }
                }
              }
            }
            n1733 = disable-structure shown="启用" {
              disable-tunnel: [w4168 w4169] -> w4098
              disable-tunnel: w4097 -> [w4166 w4169]
              frame Disabled {
                n1734 = call <vilib>:"Boolean Crossing PtByPt.vi"("direction"=enum16{"either", "false-true", "true-false"}."true-false", "input"=w4166) -> ("crossing"=w4168:bool)  [unwired: 1 in]
              }
              frame Enabled {
              }
            }
            n1735 = case shown="假" w4098 {
              frame False {
                n1736 = local write "102数据回复写入"(FALSE ("102数据回复写入")) -> ()
              }
              frame True {
              }
            }
            n1737 = call <vilib>:"Boolean Crossing PtByPt.vi"("direction"=enum16{"either", "false-true", "true-false"}."false-true", "input"=w4097) -> ("crossing"=w4135:bool)  [unwired: 1 in]
            n1738 = case shown="真" w4135 {
              tunnel: [w4174 w4188] -> w4106
              tunnel: [w4173 w4176] -> w4105
              tunnel: w4134 -> [w4173 w4190]
              tunnel: w4133 -> [w4174 w4191]
              frame False {
              }
              frame True {
                w4211 = u16 2 items=["byte", "word", "Dword"] ("数据类型")
                w4213 = u8 132 items=["I/O (P)"=128, "Input (I)"=129, "Output (Q)"=130, "Bit Memory (M)"=131, "Data (DB)"=132, "Instance Data (DI)"=133, "Local Data (L)"=134, "Predecessor Local Data (VL)"=135] ("寄存器类型")
                w4202 = u32 100 ("y")
                w4197 = u16 1 items=["byte", "word", "Dword"] ("数据类型")
                w4199 = u8 132 items=["I/O (P)"=128, "Input (I)"=129, "Output (Q)"=130, "Bit Memory (M)"=131, "Data (DB)"=132, "Instance Data (DI)"=133, "Local Data (L)"=134, "Predecessor Local Data (VL)"=135] ("寄存器类型")
                w4192 = u16 2 items=["byte", "word", "Dword"] ("数据类型")
                w4194 = u8 132 items=["I/O (P)"=128, "Input (I)"=129, "Output (Q)"=130, "Bit Memory (M)"=131, "Data (DB)"=132, "Instance Data (DI)"=133, "Local Data (L)"=134, "Predecessor Local Data (VL)"=135] ("寄存器类型")
                n1739 = call "S7_Read.vi"("TCP"=w4191, "DB #"=u16 20, "读取长度"=u16 3, "寄存器类型"=w4213, "起始地址"=u32 128, "数据类型"=w4211, "error in"=w4190) -> ("TCP"=w4234:refnum<k5>, "数据"=w4237:u32[], "error out"=w4235:errorcluster)  [unwired: 5 in, 1 out]
                n1740 = Number To Decimal String(number=w4237) -> (decimal integer string=w4236:string[])  [unwired: 1 in]
                n1741 = Index Array(array=w4236) -> (element #1=w4244:string, element #2=w4248:string, element #3=w4245:string)  [unwired: 3 in]
                n1742 = call "S7_Read.vi"("TCP"=w4234, "DB #"=u16 20, "读取长度"=u16 6, "寄存器类型"=w4194, "起始地址"=u32 60, "数据类型"=w4192, "error in"=w4235) -> ("TCP"=w4216:refnum<k5>, "数据"=w4218:u32[], "error out"=w4217:errorcluster)  [unwired: 5 in, 1 out]
                n1743 = Index Array(array=w4218) -> (element #1=w4220:u32, element #2=w4221:u32, element #3=w4223:u32, element #4=w4224:u32, element #5=w4225:u32, element #6=w4226:u32)  [unwired: 6 in]
                n1744 = Divide(x=w4221, y=w4202) -> (x/y=w4222:dbl)
                n1745 = Divide(x=w4225, y=w4202) -> (x/y=w4227:dbl)
                n1746 = Divide(x=w4226, y=w4202) -> (x/y=w4228:dbl)
                n1747 = call "S7_Read.vi"("TCP"=w4216, "DB #"=u16 20, "读取长度"=u16 2, "寄存器类型"=w4199, "起始地址"=u32 84, "数据类型"=w4197, "error in"=w4217) -> ("TCP"=w4188:refnum<k5>, "数据"=w4219:u32[], "error out"=w4187:errorcluster)  [unwired: 5 in, 1 out]
                n1748 = Number To Decimal String(number=w4220) -> (decimal integer string=w4238:string)  [unwired: 1 in]
                n1749 = Number To Fractional String(number=w4222, precision (6)=i16 2 ("精度(6)")) -> (F-format string=w4241:string)  [unwired: 2 in]
                n1750 = Number To Decimal String(number=w4223) -> (decimal integer string=w4239:string)  [unwired: 1 in]
                n1751 = Number To Decimal String(number=w4224) -> (decimal integer string=w4240:string)  [unwired: 1 in]
                n1752 = Number To Fractional String(number=w4227, precision (6)=i16 2 ("精度(6)")) -> (F-format string=w4242:string)  [unwired: 2 in]
                n1753 = Number To Fractional String(number=w4228, precision (6)=i16 2 ("精度(6)")) -> (F-format string=w4243:string)  [unwired: 2 in]
                n1754 = Index Array(array=w4219) -> (element #1=w4229:u32, element #2=w4178:u32)  [unwired: 2 in]
                n1755 = Number To Boolean Array(number=w4178) -> (Boolean array=w4179:bool[])
                n1756 = Equal?(x=w4229, y=u32 1) -> (x = y?=w4230:bool)
                n1757 = Delete From Array(array=w4179, length=8 ("长度"), index=8 ("索引")) -> (deleted portion=w4181:bool[])  [unwired: 1 out]
                n1758 = case shown="真" w4230 {
                  tunnel: ["NG" "OK"] -> w4233
                  frame False {
                  }
                  frame True {
                  }
                }
                n1759 = local read "Flange_5025570"() -> (w4247:string)
                n1760 = local read "Sleeve_5020001"() -> (w4246:string)
                n1761 = Boolean Array To Number(Boolean array=w4181) -> (number=w4180:u32)
                n1762 = Format Date/Time String(time format string (%c)="%Y-%m-%d" ("时间格式字符串(%c)")) -> (date/time string=w4231:string)  [unwired: 2 in]
                n1763 = Get Date/Time String(want seconds? (F)=TRUE ("需要秒？(F)")) -> (time string=w4232:string)  [unwired: 2 in, 1 out]
                n1764 = Insert Into Array(array=u32[] [], new element=w4180) -> (w4184:u32[])  [unwired: 1 in]
                n1765 = To Unsigned Byte Integer(number=w4184) -> (unsigned 8bit integer=w4186:u8[])
                n1766 = Byte Array To String(unsigned byte array=w4186) -> (string=w4177:string)
                n1767 = Insert Into Array(array=string[] [] ("数组"), index=0 ("索引"), new element #1="102" ("新元素/子数组"), new element #2=w4233, new element #3=w4231, new element #4=w4232, new element #5=w4233, new element #6=w4238, new element #7=w4239, new element #8=w4240, new element #9=w4241, new element #10=w4242, new element #11=w4243, new element #12=w4244, new element #13=w4248, new element #14=w4245, new element #15=w4177, new element #16=w4246, new element #17=w4247) -> (w4175:string[])
                n1768 = stacked-sequence {
                  tunnel: w4187 -> [_ w4253]
                  tunnel: [_ w4250] -> w4176
                  tunnel: w4175 -> [w4249 _]
                  frame #0 {
                    "ST102数据" <- w4249
                  }
                  frame #1 {
                    n1769 = property on="ST102数据读取（事件）" class="Bool (严格)"(error in=w4253, "Val(Sgnl)"=TRUE ("值(信号)")) -> (error out=w4251:errorcluster)  [unwired: 1 in, 1 out]
                    n1770 = disable-structure shown="禁用" {
                      disable-tunnel: w4251 -> [w4255 w4257]
                      disable-tunnel: [w4254 w4257] -> w4250
                      frame Disabled {
                        n1771 = property on="ST10画曲线" class="Bool (严格)"(error in=w4255, "Val(Sgnl)"=TRUE ("值(信号)")) -> (error out=w4254:errorcluster)  [unwired: 1 in, 1 out]
                      }
                      frame Enabled {
                      }
                    }
                  }
                }
              }
            }
            n1772 = call "S7_Read.vi"("TCP"=w4106, "DB #"=u16 20, "读取长度"=u16 15, "寄存器类型"=w4109, "起始地址"=u32 90, "数据类型"=w4107, "error in"=w4105) -> ("TCP"=w4123:refnum<k5>, "数据"=w4132:u32[], "error out"=w4122:errorcluster)  [unwired: 5 in, 1 out]
            n1773 = To Unsigned Word Integer(number=w4132) -> (unsigned 16bit integer=w4131:u16[])
            n1774 = call "还原为字符串.vi"("输入数组"=w4131) -> ("字符串"=w4129:string)  [unwired: 9 in, 1 out]
            n1775 = call "S7_Read.vi"("TCP"=w4123, "DB #"=u16 20, "读取长度"=u16 15, "寄存器类型"=w4116, "起始地址"=u32 110, "数据类型"=w4114, "error in"=w4122) -> ("TCP"=w4104:refnum<k5>, "数据"=w4124:u32[], "error out"=w4103:errorcluster)  [unwired: 5 in, 1 out]
            n1776 = To Unsigned Word Integer(number=w4124) -> (unsigned 16bit integer=w4125:u16[])
            n1777 = Match Pattern(string=w4129, regular expression="\r" ("正则表达式")) -> (before substring=w4130:string)  [unwired: 1 in, 3 out]
            n1778 = call "还原为字符串.vi"("输入数组"=w4125) -> ("字符串"=w4127:string)  [unwired: 9 in, 1 out]
            n1779 = Match Pattern(string=w4130, regular expression="\u0000" ("正则表达式")) -> (before substring=→"Sleeve_5020001":string)  [unwired: 1 in, 3 out]
            n1780 = Match Pattern(string=w4127, regular expression="\r" ("正则表达式")) -> (before substring=w4126:string)  [unwired: 1 in, 3 out]
            n1781 = Match Pattern(string=w4126, regular expression="\u0000" ("正则表达式")) -> (before substring=→"Flange_5025570":string)  [unwired: 1 in, 3 out]
          }
          frame "写" {
            w4321 = u8 132 items=["I/O (P)"=128, "Input (I)"=129, "Output (Q)"=130, "Bit Memory (M)"=131, "Data (DB)"=132, "Instance Data (DI)"=133, "Local Data (L)"=134, "Predecessor Local Data (VL)"=135] ("寄存器类型")
            w4322 = u16 1 items=["byte", "word", "Dword"] ("数据类型")
            w4331 = u8 132 items=["I/O (P)"=128, "Input (I)"=129, "Output (Q)"=130, "Bit Memory (M)"=131, "Data (DB)"=132, "Instance Data (DI)"=133, "Local Data (L)"=134, "Predecessor Local Data (VL)"=135] ("寄存器类型")
            w4332 = u16 1 items=["byte", "word", "Dword"] ("数据类型")
            w4336 = u8 132 items=["I/O (P)"=128, "Input (I)"=129, "Output (Q)"=130, "Bit Memory (M)"=131, "Data (DB)"=132, "Instance Data (DI)"=133, "Local Data (L)"=134, "Predecessor Local Data (VL)"=135] ("寄存器类型")
            w4335 = u16 1 items=["byte", "word", "Dword"] ("数据类型")
            w4346 = u8 132 items=["I/O (P)"=128, "Input (I)"=129, "Output (Q)"=130, "Bit Memory (M)"=131, "Data (DB)"=132, "Instance Data (DI)"=133, "Local Data (L)"=134, "Predecessor Local Data (VL)"=135] ("寄存器类型")
            w4343 = u16 1 items=["byte", "word", "Dword"] ("数据类型")
            n1782 = local read "10看门狗"() -> (w4341:i32)
            n1783 = case shown="0" w4341 {
              tunnel: [0 ("y") 1 ("y")] -> w4347
              frame 1, Default {
              }
              frame 0 {
              }
            }
            "10看门狗" <- w4347
            n1784 = call "S7_Write.vi"("TCP"=w4342, "寄存器类型"=w4346, "DB #"=u16 20, "写入地址"=u32 2, "数据类型"=w4343, "写入数据"=w4347) -> ("TCP"=w4340:refnum<k5>, "error out"=w4339:errorcluster)  [unwired: 7 in, 1 out]
            n1785 = case shown="真" "101扫码回复写入" {
              tunnel: [999 w4401] -> w4334
              frame False {
              }
              frame True {
                n1786 = local read "扫码请求回复101"() -> (w4402:string)
                n1787 = Decimal String To Number(string=w4402) -> (number=w4401:i32)  [unwired: 2 in, 1 out]
              }
            }
            n1788 = call "S7_Write.vi"("TCP"=w4340, "寄存器类型"=w4336, "DB #"=u16 20, "写入地址"=u32 4, "数据类型"=w4335, "写入数据"=w4334, "error in"=w4339) -> ("TCP"=w4326:refnum<k5>, "error out"=w4325:errorcluster)  [unwired: 6 in, 1 out]
            n1789 = case shown="真" "102扫码回复写入" {
              tunnel: [999 w4397] -> w4327
              tunnel: w4326 -> [w4374 w4391]
              tunnel: w4325 -> [w4373 w4390]
              tunnel: [w4374 w4377] -> w4324
              tunnel: [w4373 w4376] -> w4323
              frame False {
              }
              frame True {
                w4384 = u8 132 items=["I/O (P)"=128, "Input (I)"=129, "Output (Q)"=130, "Bit Memory (M)"=131, "Data (DB)"=132, "Instance Data (DI)"=133, "Local Data (L)"=134, "Predecessor Local Data (VL)"=135] ("寄存器类型")
                w4385 = u16 1 items=["byte", "word", "Dword"] ("数据类型")
                w4393 = u8 132 items=["I/O (P)"=128, "Input (I)"=129, "Output (Q)"=130, "Bit Memory (M)"=131, "Data (DB)"=132, "Instance Data (DI)"=133, "Local Data (L)"=134, "Predecessor Local Data (VL)"=135] ("寄存器类型")
                w4392 = u16 1 items=["byte", "word", "Dword"] ("数据类型")
                n1790 = local read "上一站号(10)"() -> (w4389:string)
                n1791 = Decimal String To Number(string=w4389) -> (number=w4388:i32)  [unwired: 2 in, 1 out]
                n1792 = call "S7_Write.vi"("TCP"=w4391, "寄存器类型"=w4393, "DB #"=u16 20, "写入地址"=u32 8, "数据类型"=w4392, "写入数据"=w4388, "error in"=w4390) -> ("TCP"=w4380:refnum<k5>, "error out"=w4381:errorcluster)  [unwired: 6 in, 1 out]
                n1793 = local read "上一站结果(10)"() -> (w4379:string)
                n1794 = Equal?(x=w4379, y="OK") -> (x = y?=w4387:bool)
                n1795 = case shown="假" w4387 {
                  tunnel: [u32 2 ("写入数据") u32 1 ("写入数据")] -> w4378
                  frame False {
                  }
                  frame True {
                  }
                }
                n1796 = local read "扫码请求回复102"() -> (w4396:string)
                n1797 = call "S7_Write.vi"("TCP"=w4380, "寄存器类型"=w4384, "DB #"=u16 20, "写入地址"=u32 10, "数据类型"=w4385, "写入数据"=w4378, "error in"=w4381) -> ("TCP"=w4377:refnum<k5>, "error out"=w4376:errorcluster)  [unwired: 6 in, 1 out]
                n1798 = Decimal String To Number(string=w4396) -> (number=w4397:i32)  [unwired: 2 in, 1 out]
              }
            }
            n1799 = call "S7_Write.vi"("TCP"=w4324, "寄存器类型"=w4331, "DB #"=u16 20, "写入地址"=u32 6, "数据类型"=w4332, "写入数据"=w4327, "error in"=w4323) -> ("TCP"=w4317:refnum<k5>, "error out"=w4318:errorcluster)  [unwired: 6 in, 1 out]
            n1800 = case shown="真" "102数据回复写入" {
              tunnel: [999 w4372] -> w4315
              frame False {
              }
              frame True {
                n1801 = local read "数据保存请求回复102"() -> (w4371:string)
                n1802 = Decimal String To Number(string=w4371) -> (number=w4372:i32)  [unwired: 2 in, 1 out]
              }
            }
            n1803 = call "S7_Write.vi"("TCP"=w4317, "寄存器类型"=w4321, "DB #"=u16 20, "写入地址"=u32 12, "数据类型"=w4322, "写入数据"=w4315, "error in"=w4318) -> ("TCP"=w4312:refnum<k5>, "error out"=w4314:errorcluster)  [unwired: 6 in, 1 out]
            n1804 = disable-structure shown="启用" {
              disable-tunnel: w4312 -> [w4350 w4360]
              disable-tunnel: [w4350 w4365] -> w4311
              disable-tunnel: w4314 -> [w4351 w4356]
              disable-tunnel: [w4351 w4364] -> w4313
              frame Disabled {
              }
              frame Enabled {
                w4361 = u16 20 ("DB #")
                w4359 = u8 132 items=["I/O (P)"=128, "Input (I)"=129, "Output (Q)"=130, "Bit Memory (M)"=131, "Data (DB)"=132, "Instance Data (DI)"=133, "Local Data (L)"=134, "Predecessor Local Data (VL)"=135] ("寄存器类型")
                w4357 = u16 1 items=["byte", "word", "Dword"] ("数据类型")
                n1805 = call "S7_Read.vi"("TCP"=w4360, "DB #"=w4361, "读取长度"=u16 1, "寄存器类型"=w4359, "起始地址"=u32 140, "数据类型"=w4357, "error in"=w4356) -> ("TCP"=w4355:refnum<k5>, "数据"=w4353:u32[], "error out"=w4354:errorcluster)  [unwired: 5 in, 1 out]
                n1806 = Index Array(array=w4353) -> (element=w4352:u32)  [unwired: 1 in]
                n1807 = case shown="1" w4352 {
                  tunnel: ["未选择" "LF37G" "LF37.1G"] -> w4363
                  frame 0, Default {
                  }
                  frame 1 {
                  }
                  frame 2 {
                  }
                }
                "产品型号10" <- w4363
                n1808 = call "S7_Write.vi"("TCP"=w4355, "寄存器类型"=w4359, "DB #"=w4361, "写入地址"=u32 142, "数据类型"=w4357, "写入数据"=w4352, "error in"=w4354) -> ("TCP"=w4365:refnum<k5>, "error out"=w4364:errorcluster)  [unwired: 6 in, 1 out]
              }
            }
          }
          frame "错误" {
            n1809 = call "S7_Close.vi"("TCP Connection Ref"=w4407) -> ("error out"=w4408:errorcluster)  [unwired: 10 in]
            n1810 = call <vilib>:"Clear Errors.vi"("error in (no error)"=w4408) -> ()  [unwired: 5 in, 2 out]
          }
          frame "退出" {
            n1811 = call "S7_Close.vi"("TCP Connection Ref"=w4414) -> ("error out"=w4415:errorcluster)  [unwired: 10 in]
            n1812 = call <vilib>:"Clear Errors.vi"("error in (no error)"=w4415) -> ()  [unwired: 5 in, 2 out]
          }
        }
      }
      n1813 = while {
        shift-right: [w708] -> _
        shift-left: errorcluster {"status"=FALSE, "code"=0, "source"=""} ("错误常量") -> [w711]
        shift-right: [w707] -> _
        shift-left: enum16{"初始化", "读", "写", "错误", "退出"}."初始化" -> [w712]
        shift-right: [w709] -> _
        shift-left: _ -> [w706]
        stop <- w705 stop-if-true
        n1814 = local read "退出"() -> (w713:bool)
        n1815 = case shown="假" w713 {
          tunnel: w712 -> [w714 _]
          tunnel: [w715 enum16{"初始化", "读", "写", "错误", "退出"}."退出"] -> w704
          tunnel: w711 -> [w716 _]
          frame False {
            n1816 = case shown="错误" w716 {
              tunnel: [w717 enum16{"初始化", "读", "写", "错误", "退出"}."错误"] -> w715
              tunnel: w714 -> [w717 _]
              frame No Error {
              }
              frame Error {
              }
            }
          }
          frame True {
          }
        }
        n1817 = Wait (ms)(milliseconds to wait=u32 80 ("等待时间（毫秒）")) -> ()  [unwired: 1 out]
        n1818 = case shown="\"写\"" w704 {
          tunnel: [w722 w742 w836 refnum<k5> refnum ("TCP") refnum<k5> refnum ("TCP")] -> w709
          tunnel: [w720 w741 w834 errorcluster {"status"=FALSE, "code"=0, "source"=""} ("error out") errorcluster {"status"=FALSE, "code"=0, "source"=""} ("error out")] -> w708
          tunnel: [enum16{"初始化", "读", "写", "错误", "退出"}."读" enum16{"初始化", "读", "写", "错误", "退出"}."写" enum16{"初始化", "读", "写", "错误", "退出"}."读" enum16{"初始化", "读", "写", "错误", "退出"}."初始化" enum16{"初始化", "读", "写", "错误", "退出"}."退出"] -> w707
          tunnel: w706 -> [_ w756 w858 w911 w918]
          tunnel: [FALSE FALSE FALSE FALSE TRUE] -> w705
          frame "初始化", Default {
            w731 = u16 0 items=["byte", "word", "Dword"] ("数据类型")
            w729 = u8 132 items=["I/O (P)"=128, "Input (I)"=129, "Output (Q)"=130, "Bit Memory (M)"=131, "Data (DB)"=132, "Instance Data (DI)"=133, "Local Data (L)"=134, "Predecessor Local Data (VL)"=135] ("寄存器类型")
            w737 = u8 0 items=["S7-1200.200.200SMART"=0, "S7-300"=2, "S7-400"=3] ("PLC 系列")
            n1819 = call "S7_Open.vi"("IP 地址"="192.168.1.80", "PLC 系列"=w737, "超时（MS）"=100) -> ("TCP"=w723:refnum<k5>, "error out"=w721:errorcluster)  [unwired: 10 in, 1 out]
            n1820 = call "S7_Read.vi"("TCP"=w723, "DB #"=u16 20, "读取长度"=u16 13, "寄存器类型"=w729, "起始地址"=u32 6, "数据类型"=w731, "error in"=w721) -> ("TCP"=w722:refnum<k5>, "数据"=w726:u32[], "error out"=w724:errorcluster)  [unwired: 5 in, 1 out]
            n1821 = To Unsigned Word Integer(number=w726) -> (unsigned 16bit integer=w725:u16[])
            n1822 = call "还原为字符串.vi"("error in (no error)"=w724, "输入数组"=w725) -> ("error out"=w720:errorcluster, "字符串"=w732:string)  [unwired: 8 in]
            n1823 = local write "80二维码"(w732) -> ()
            n1824 = case shown="错误" w720 {
              tunnel: [FALSE TRUE] -> w733
              frame No Error {
              }
              frame Error {
              }
            }
            n1825 = local write "ST80通讯状态"(w733) -> ()
          }
          frame "读" {
            w757 = u16 0 items=["byte", "word", "Dword"] ("数据类型")
            w759 = u8 132 items=["I/O (P)"=128, "Input (I)"=129, "Output (Q)"=130, "Bit Memory (M)"=131, "Data (DB)"=132, "Instance Data (DI)"=133, "Local Data (L)"=134, "Predecessor Local Data (VL)"=135] ("寄存器类型")
            n1826 = call "S7_Read.vi"("TCP"=w756, "DB #"=u16 20, "读取长度"=u16 1, "寄存器类型"=w759, "起始地址"=u32 0, "数据类型"=w757) -> ("TCP"=w754:refnum<k5>, "数据"=w764:u32[], "读取成功"=w767:bool, "error out"=w753:errorcluster)  [unwired: 6 in]
            n1827 = Not(x=w767) -> (.not. x?=→"ST80通讯状态":bool)
            n1828 = Index Array(array=w764, index=0 ("索引")) -> (element=w765:u32)
            n1829 = Number To Boolean Array(number=w765) -> (Boolean array=w766:bool[])
            n1830 = Index Array(array=w766, index #1=0 ("索引")) -> (element #1=w746:bool, element #2=w743:bool)  [unwired: 1 in]
            "ST80扫码请求" <- w746
            "ST80数据保存请求" <- w743
            n1831 = disable-structure shown="启用" {
              disable-tunnel: w746 -> [w771 w773]
              disable-tunnel: [w770 w773] -> w744
              frame Disabled {
                n1832 = call <vilib>:"Boolean Crossing PtByPt.vi"("direction"=enum16{"either", "false-true", "true-false"}."true-false", "input"=w771) -> ("crossing"=w770:bool)  [unwired: 1 in]
